vi "global-Report.vi"() -> ()   [LabVIEW 2015]
panel:
  out "报警-50":bool[](array[boolean])
  out "报警-40":bool[](array[boolean])
  out "报警-30":bool[](array[boolean])
  out "报警-20":bool[](array[boolean])
  out "报警-10":bool[](array[boolean])
  out "报警-继保":bool[](array[boolean])
  in  "报警-管理机":bool[](array[boolean])
  out "报告-50":bool[](array[boolean])
  out "报告-40":bool[](array[boolean])
  out "报告-30":bool[](array[boolean])
  out "报告-20":bool[](array[boolean])
  out "报告-10":bool[](array[boolean])
  out "报告-继保":bool[](array[boolean])
  out "报告-管理机":bool[](array[boolean])
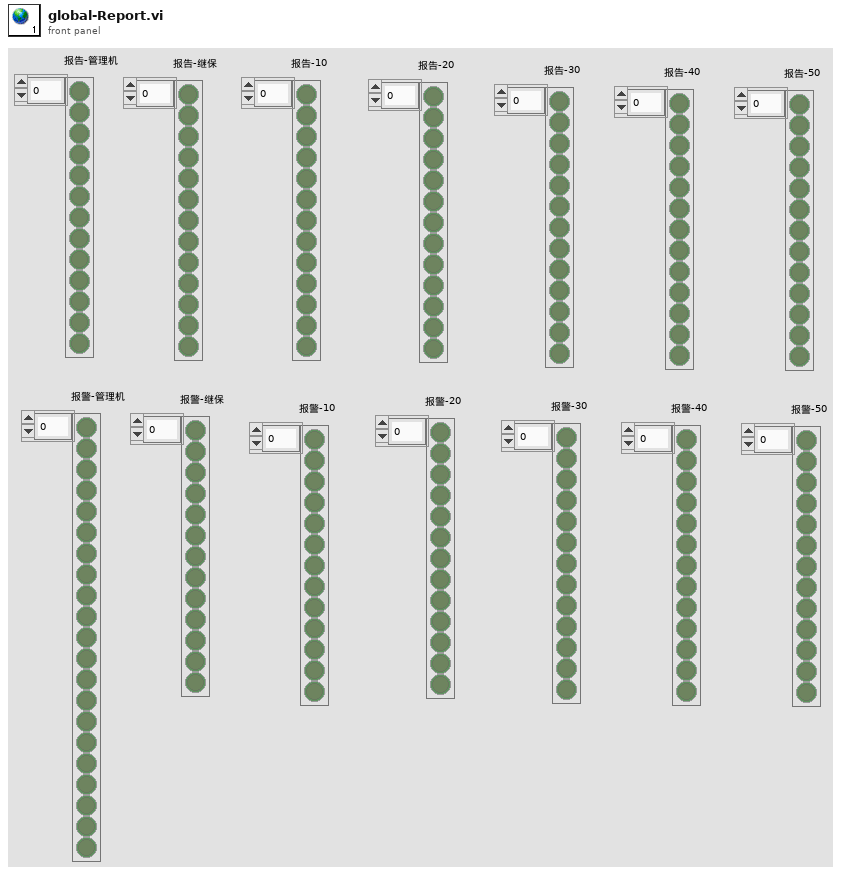
[diagram p1: front panel]
diagram:
